vi "Path to Game Controller Settings Polymorphic.vi"(6 "File Path":path, 8 "error in (no error)":errorcluster, 10 "XML Elements":string) -> (0 "error out":errorcluster, 1 "File Path Out":path)   [LabVIEW 2014]
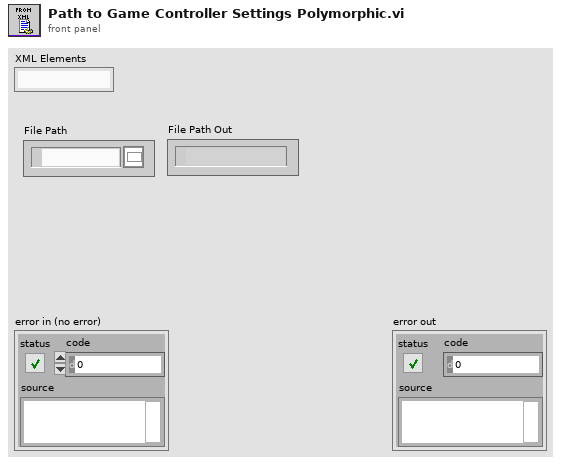
[diagram p1: front panel]
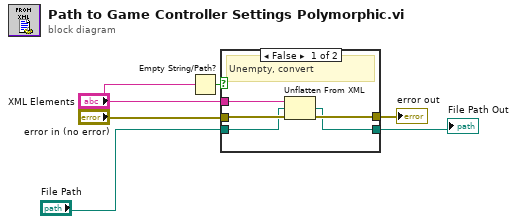
[diagram p0: block diagram]
diagram:
  n1 = Empty String/Path?(string/path="XML Elements") -> (empty?=w3:bool)
  n2 = case shown="False" w3 {
    tunnel: "error in (no error)" -> [w11 w12]
    tunnel: "File Path" -> [w8 w13]
    tunnel: [w7 w13] -> w2
    tunnel: [w10 w12] -> w5
    tunnel: "XML Elements" -> [w9 _]
    frame False {
      # "Unempty, convert"
      n3 = Unflatten From XML(xml string=w9, type=w8, error in (no error)=w11) -> (value=w7:path, error out=w10:errorcluster)
    }
    frame True {
      # "Empty, default values"
    }
  }
  "error out" <- w5
  "File Path Out" <- w2
